vi "FT_Search All Select description.vi"(8 "error in (no error)":errorcluster, 11 "CTA Test#":string="CTA013A") -> (0 "error Out":errorcluster, 2 "All FT":T1(array[cluster]), 3 "Select Ft":T2)   [LabVIEW 2019]
uses:
  FT_Search all (state machine).ctl
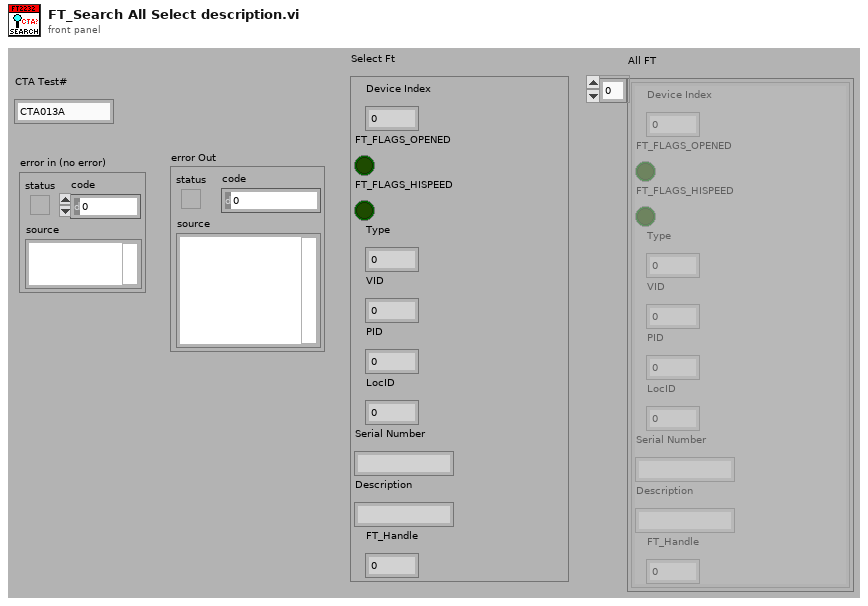
[diagram p1: front panel]
types:
  T1 = cluster{"Device Index":u32, "FT_FLAGS_OPENED":bool, "FT_FLAGS_HISPEED":bool, "Type":u32, "VID":u32, "PID":u32, "LocID":i32, "Serial Number":string, "Description":string, "FT_Handle":u32}[]
  T2 = cluster{"Device Index":u32, "FT_FLAGS_OPENED":bool, "FT_FLAGS_HISPEED":bool, "Type":u32, "VID":u32, "PID":u32, "LocID":i32, "Serial Number":string, "Description":string, "FT_Handle":u32}
  T3 = typedef "FT_Search all (state machine).ctl" = enum16{"Init", "Re_scan", "Close if Open", "Open FT", "Report FT", "Exit", "Error"}
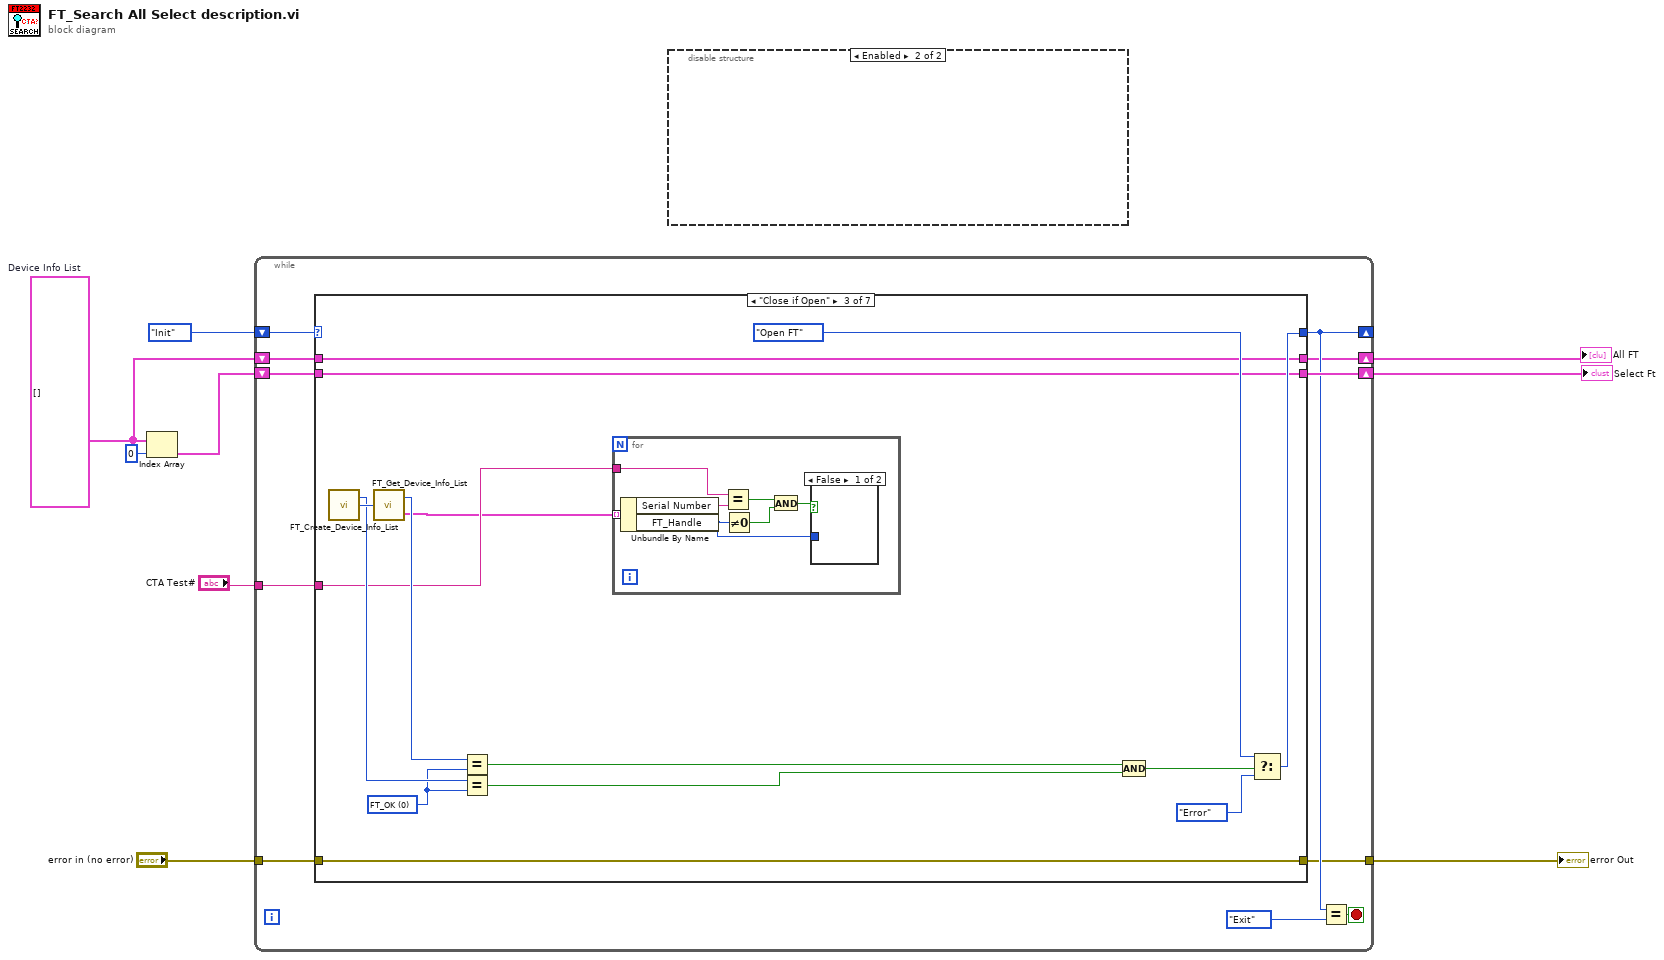
[diagram p0: block diagram]
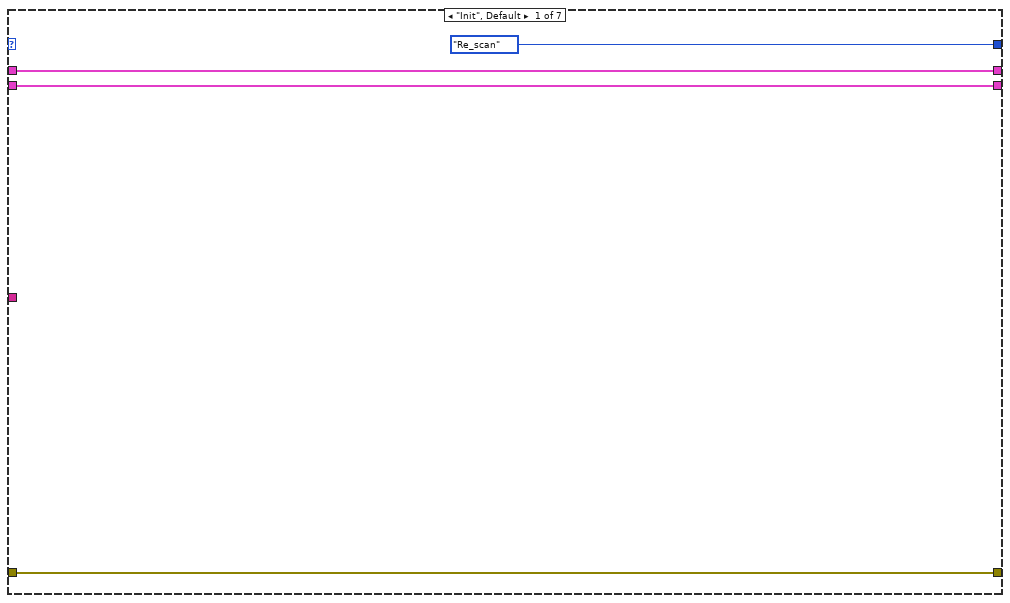
[diagram p3: hidden frame]
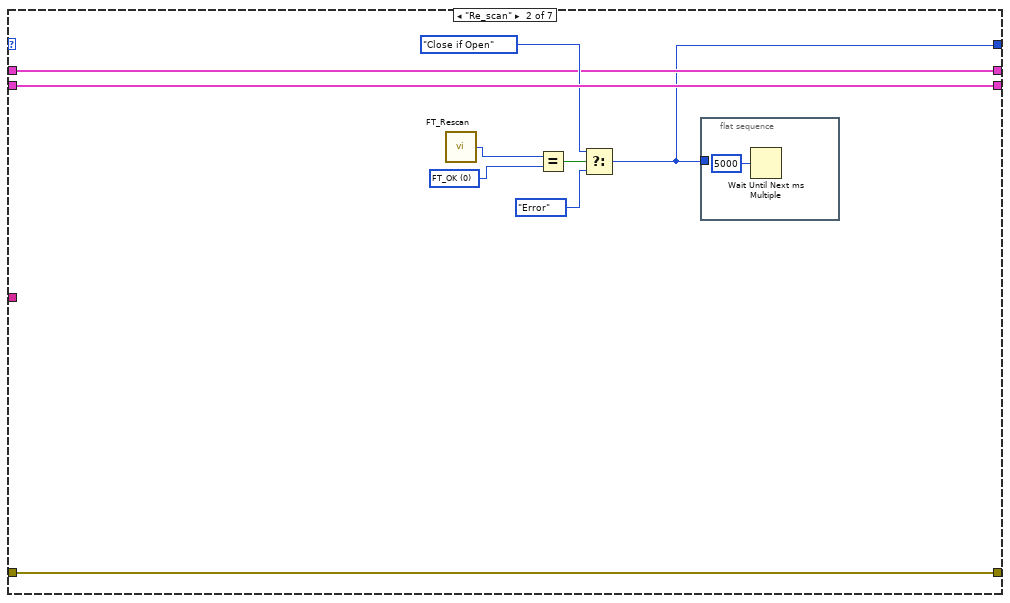
[diagram p4: hidden frame]
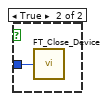
[diagram p5: hidden frame]
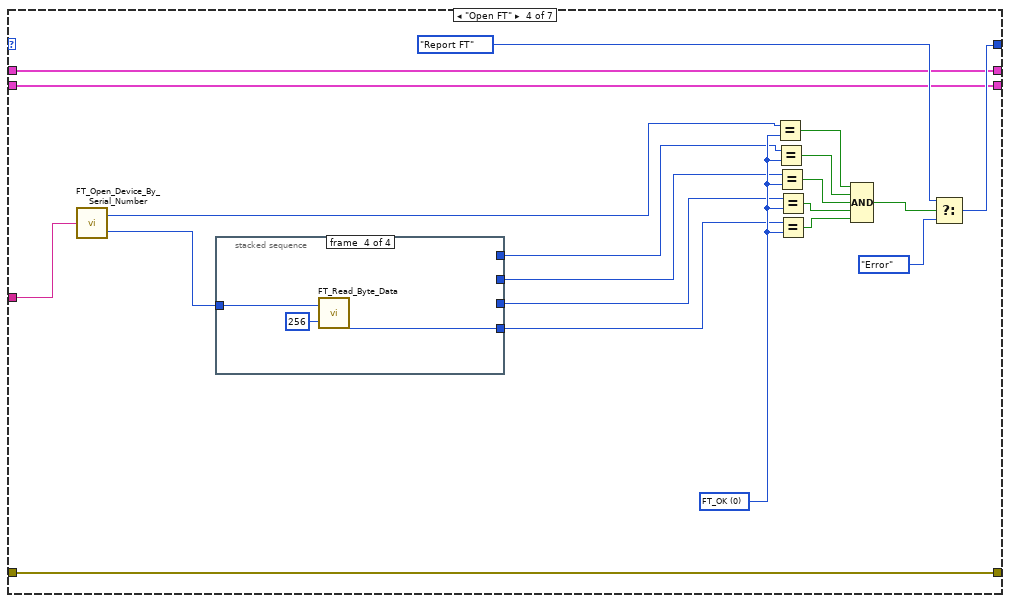
[diagram p6: hidden frame]
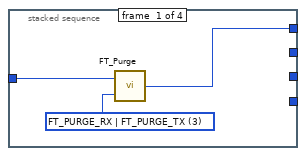
[diagram p7: hidden frame]
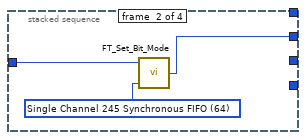
[diagram p8: hidden frame]
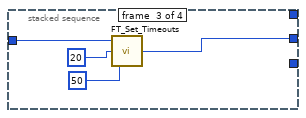
[diagram p9: hidden frame]
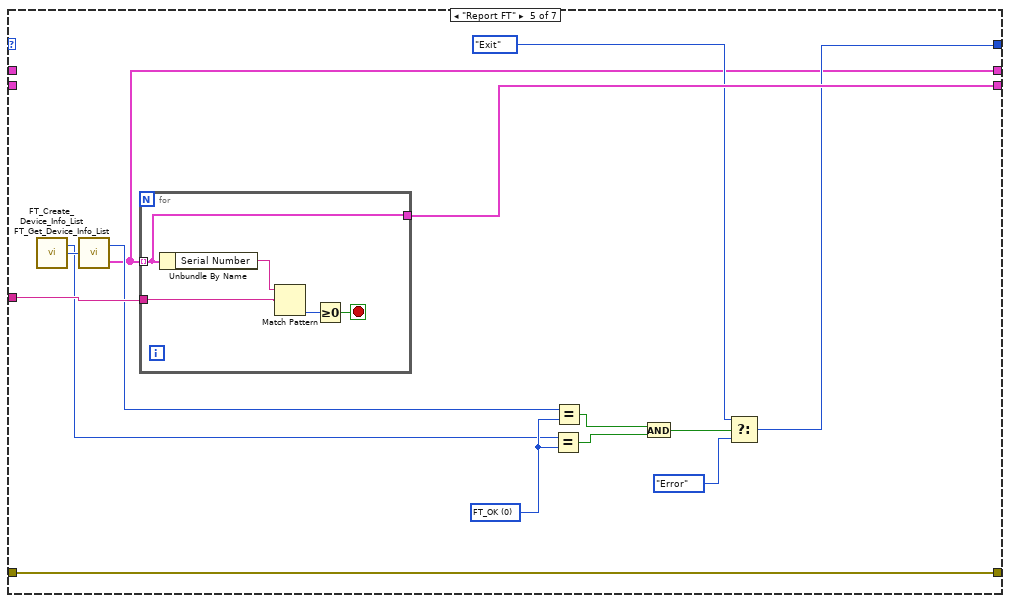
[diagram p10: hidden frame]
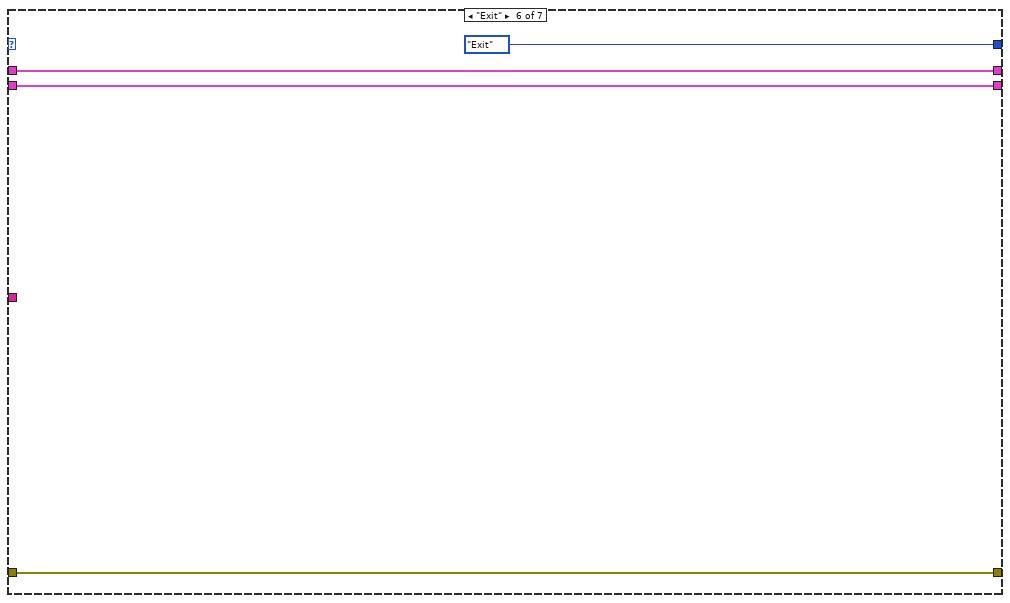
[diagram p11: hidden frame]
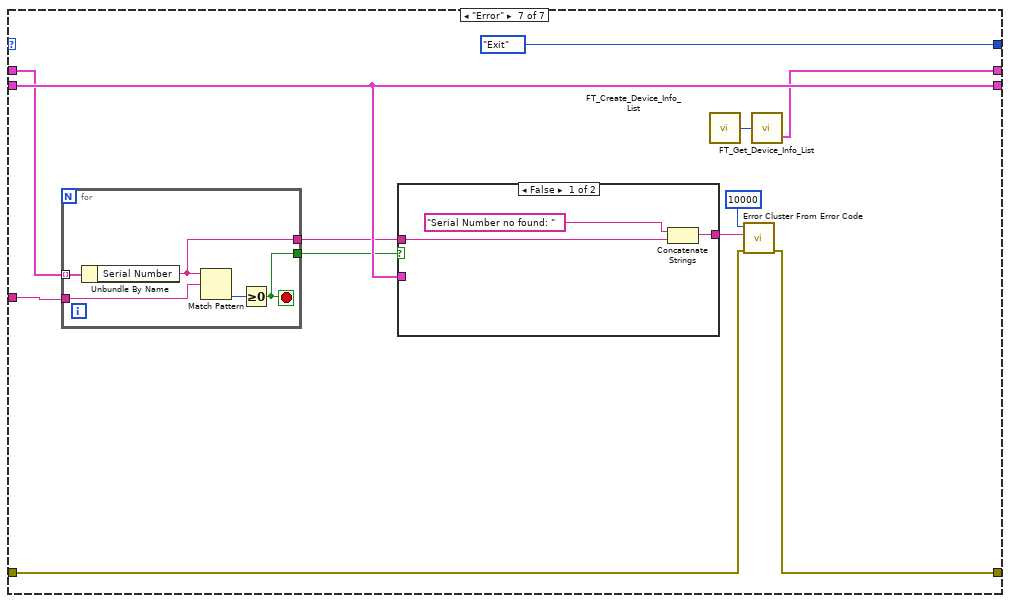
[diagram p12: hidden frame]
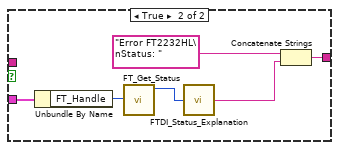
[diagram p13: hidden frame]
diagram:
  w3 = T1 []  # Device Info List
  n1 = Index Array(array=w3, index=0) -> (element=w6:T2)
  n2 = while {
    shift-right: [w15] -> _
    shift-left: FT_Search_all_(state_machine)."Init" ("State Search FT") -> [w20]
    tunnel: "CTA Test#" -> [w19]
    shift-right: [w16] -> w5
    shift-left: w6 -> [w18]
    tunnel: "error in (no error)" -> [w17]
    tunnel: [w12] -> w4
    shift-right: [w11] -> w2
    shift-left: w3 -> [w10]
    stop <- w13 stop-if-true
    n3 = case shown="\"Error\"" w20 {
      tunnel: w19 -> [_ _ w38 w65 w103 _ w118]
      tunnel: w18 -> [w24 w33 w35 w58 _ w113 w124]
      tunnel: w17 -> [w22 w32 w48 w77 w101 w111 w121]
      tunnel: [w24 w33 w35 w58 w102 w113 w124] -> w16
      tunnel: [FT_Search_all_(state_machine)."Re_scan" ("State Search FT") w25 w39 w67 w92 FT_Search_all_(state_machine)."Exit" ("State Search FT") FT_Search_all_(state_machine)."Exit" ("State Search FT")] -> w15
      tunnel: [w22 w32 w48 w77 w101 w111 w120] -> w12
      tunnel: [w21 w26 w37 w66 w91 w110 w114] -> w11
      tunnel: w10 -> [w21 w26 w37 w66 _ w110 w119]
      frame "Init", Default {
      }
      frame "Re_scan" {
        w31 = u32 0 items=["FT_OK", "FT_INVALID_HANDLE", "FT_DEVICE_NOT_FOUND", "FT_DEVICE_NOT_OPENED", "FT_IO_ERROR", "FT_INSUFFICIENT_RESOURCES", "FT_INVALID_PARAMETER", "FT_INVALID_BAUD_RATE", "FT_DEVICE_NOT_OPENED_FOR_ERASE", "FT_DEVICE_NOT_OPENED_FOR_WRITE", "FT_FAILED_TO_WRITE_DEVICE", "FT_EEPROM_READ_FAILED", "FT_EEPROM_WRITE_FAILED", "FT_EEPROM_ERASE_FAILED", "FT_EEPROM_NOT_PRESENT", "FT_EEPROM_NOT_PROGRAMMED", "FT_INVALID_ARGS", "FT_NOT_SUPPORTED", "FT_OTHER_ERROR"] ("FT_Status")
        n4 = call "FT_Rescan.vi"() -> ("FT_Status"=w30:u32)  [unwired: 1 in]
        n5 = Equal?(x=w30, y=w31) -> (x = y?=w29:bool)
        n6 = Select(t=FT_Search_all_(state_machine)."Close if Open" ("State Search FT"), s=w29, f=FT_Search_all_(state_machine)."Error") -> (s? t:f=w25:T3)
        n7 = flat-sequence {
          tunnel: w25 -> [_]
          frame #0 {
            n8 = Wait Until Next ms Multiple(millisecond multiple=u32 5000) -> ()  [unwired: 1 out]
          }
        }
      }
      frame "Close if Open" {
        w44 = u32 0 items=["FT_OK", "FT_INVALID_HANDLE", "FT_DEVICE_NOT_FOUND", "FT_DEVICE_NOT_OPENED", "FT_IO_ERROR", "FT_INSUFFICIENT_RESOURCES", "FT_INVALID_PARAMETER", "FT_INVALID_BAUD_RATE", "FT_DEVICE_NOT_OPENED_FOR_ERASE", "FT_DEVICE_NOT_OPENED_FOR_WRITE", "FT_FAILED_TO_WRITE_DEVICE", "FT_EEPROM_READ_FAILED", "FT_EEPROM_WRITE_FAILED", "FT_EEPROM_ERASE_FAILED", "FT_EEPROM_NOT_PRESENT", "FT_EEPROM_NOT_PROGRAMMED", "FT_INVALID_ARGS", "FT_NOT_SUPPORTED", "FT_OTHER_ERROR"] ("FT_Status")
        n9 = call "FT_Create_Device_Info_List.vi"() -> ("Number of Devices"=w49:u32, "FT_Status"=w46:u32)
        n10 = call "FT_Get_Device_Info_List.vi"("Number Of Devices"=w49) -> ("FT_Status"=w45:u32, "Device Info List"=w36:T1)
        n11 = Equal?(x=w45, y=w44) -> (x = y?=w43:bool)
        n12 = Equal?(x=w46, y=w44) -> (x = y?=w42:bool)
        n13 = for {
          tunnel: w36 -> [w56] mode=indexing
          tunnel: w38 -> [w55]
          n14 = Unbundle By Name(w56) -> ("Serial Number"=w50:string, "FT_Handle"=w51:u32)
          n15 = Equal?(x=w55, y=w50) -> (x = y?=w53:bool)
          n16 = Not Equal To 0?(x=w51) -> (x != 0?=w54:bool)
          n17 = And(x=w53, y=w54) -> (x .and. y?=w52:bool)
          n18 = case shown="False" w52 {
            tunnel: w51 -> [_ w57]
            frame False {
            }
            frame True {
              n19 = call "FT_Close_Device.vi"("Handle"=w57) -> ()  [unwired: 1 out]
            }
          }
        }
        n20 = Compound Arithmetic op=AND(w43, w42) -> (w41:bool)
        n21 = Select(t=FT_Search_all_(state_machine)."Open FT" ("State Search FT"), s=w41, f=FT_Search_all_(state_machine)."Error") -> (s? t:f=w39:T3)
      }
      frame "Open FT" {
        w76 = u32 0 items=["FT_OK", "FT_INVALID_HANDLE", "FT_DEVICE_NOT_FOUND", "FT_DEVICE_NOT_OPENED", "FT_IO_ERROR", "FT_INSUFFICIENT_RESOURCES", "FT_INVALID_PARAMETER", "FT_INVALID_BAUD_RATE", "FT_DEVICE_NOT_OPENED_FOR_ERASE", "FT_DEVICE_NOT_OPENED_FOR_WRITE", "FT_FAILED_TO_WRITE_DEVICE", "FT_EEPROM_READ_FAILED", "FT_EEPROM_WRITE_FAILED", "FT_EEPROM_ERASE_FAILED", "FT_EEPROM_NOT_PRESENT", "FT_EEPROM_NOT_PROGRAMMED", "FT_INVALID_ARGS", "FT_NOT_SUPPORTED", "FT_OTHER_ERROR"] ("FT_Status")
        n22 = call "FT_Open_Device_By_Serial_Number.vi"("Device Serial Number"=w65) -> ("FT_Status"=w63:u32, "Handle"=w64:u32)
        n23 = stacked-sequence {
          tunnel: w64 -> [w80 w82 w85 w90]
          tunnel: [w78 _ _ _] -> w62
          tunnel: [_ w81 _ _] -> w61
          tunnel: [_ _ w84 _] -> w60
          tunnel: [_ _ _ w88] -> w59
          frame #0 {
            w79 = u32 3 items=["FT_PURGE_RX"=1, "FT_PURGE_TX"=2, "FT_PURGE_RX | FT_PURGE_TX"=3] ("Purge Flags")
            n24 = call "FT_Purge.vi"("Purge Flags"=w79, "Handle"=w80) -> ("FT_Status"=w78:u32)
          }
          frame #1 {
            w83 = u8 64 items=["Reset Bit Mode"=0, "Asynchronous Bit Bang"=1, "MPSSE"=2, "Synchronous Bit Bang"=4, "MCU Host Bus Emulation"=8, "Fast Opto-Isolated Serial"=16, "CBUS Bit Bang"=32, "Single Channel 245 Synchronous FIFO"=64] ("Bit Mode")
            n25 = call "FT_Set_Bit_Mode.vi"("Bit Mode"=w83, "Handle"=w82) -> ("FT_Status"=w81:u32)  [unwired: 1 in]
          }
          frame #2 {
            n26 = call "FT_Set_Timeouts.vi"("Write Timeout"=u32 50, "Read Timeout"=u32 20, "Handle"=w85) -> ("FT_Status"=w84:u32)
          }
          frame #3 {
            n27 = call "FT_Read_Byte_Data.vi"("Handle"=w90, "Bytes To Read"=u32 256) -> ("FT_Status"=w88:u32)  [unwired: 2 out]
          }
        }
        n28 = Equal?(x=w63, y=w76) -> (x = y?=w75:bool)
        n29 = Equal?(x=w62, y=w76) -> (x = y?=w74:bool)
        n30 = Equal?(x=w61, y=w76) -> (x = y?=w73:bool)
        n31 = Equal?(x=w60, y=w76) -> (x = y?=w72:bool)
        n32 = Equal?(x=w59, y=w76) -> (x = y?=w71:bool)
        n33 = Compound Arithmetic op=AND(w75, w74, w73, w72, w71) -> (w69:bool)
        n34 = Select(t=FT_Search_all_(state_machine)."Report FT" ("State Search FT"), s=w69, f=FT_Search_all_(state_machine)."Error") -> (s? t:f=w67:T3)
      }
      frame "Report FT" {
        w100 = u32 0 items=["FT_OK", "FT_INVALID_HANDLE", "FT_DEVICE_NOT_FOUND", "FT_DEVICE_NOT_OPENED", "FT_IO_ERROR", "FT_INSUFFICIENT_RESOURCES", "FT_INVALID_PARAMETER", "FT_INVALID_BAUD_RATE", "FT_DEVICE_NOT_OPENED_FOR_ERASE", "FT_DEVICE_NOT_OPENED_FOR_WRITE", "FT_FAILED_TO_WRITE_DEVICE", "FT_EEPROM_READ_FAILED", "FT_EEPROM_WRITE_FAILED", "FT_EEPROM_ERASE_FAILED", "FT_EEPROM_NOT_PRESENT", "FT_EEPROM_NOT_PROGRAMMED", "FT_INVALID_ARGS", "FT_NOT_SUPPORTED", "FT_OTHER_ERROR"] ("FT_Status")
        n35 = call "FT_Create_Device_Info_List.vi"() -> ("Number of Devices"=w104:u32, "FT_Status"=w99:u32)
        n36 = call "FT_Get_Device_Info_List.vi"("Number Of Devices"=w104) -> ("FT_Status"=w98:u32, "Device Info List"=w91:T1)
        n37 = for {
          tunnel: w91 -> [w105] mode=indexing
          tunnel: w103 -> [w107]
          tunnel: [w105] -> w102
          stop <- w106 stop-if-true
          n38 = Unbundle By Name(w105) -> ("Serial Number"=w108:string)
          n39 = Match Pattern(string=w108, regular expression=w107) -> (offset past match=w109:i32)  [unwired: 4 out]
          n40 = Greater Or Equal To 0?(x=w109) -> (x >= 0?=w106:bool)
        }
        n41 = Equal?(x=w99, y=w100) -> (x = y?=w96:bool)
        n42 = Equal?(x=w98, y=w100) -> (x = y?=w97:bool)
        n43 = And(x=w97, y=w96) -> (x .and. y?=w94:bool)
        n44 = Select(t=FT_Search_all_(state_machine)."Exit" ("State Search FT"), s=w94, f=FT_Search_all_(state_machine)."Error") -> (s? t:f=w92:T3)
      }
      frame "Exit" {
      }
      frame "Error" {
        n45 = for {
          tunnel: w119 -> [w138] mode=indexing
          tunnel: w118 -> [w137]
          tunnel: [w136] -> w117
          tunnel: [w135] -> w116
          stop <- w136 stop-if-true
          n46 = Unbundle By Name(w138) -> ("Serial Number"=w135:string)
          n47 = Match Pattern(string=w135, regular expression=w137) -> (offset past match=w139:i32)  [unwired: 4 out]
          n48 = Greater Or Equal To 0?(x=w139) -> (x >= 0?=w136:bool)
        }
        n49 = case shown="False" w117 {
          tunnel: w124 -> [_ w134]
          tunnel: [w128 w130] -> w122
          tunnel: w116 -> [w126 _]
          frame False {
            n50 = Concatenate Strings("Serial Number no found: ", w126) -> (w128:string)
          }
          frame True {
            n51 = Unbundle By Name(w134) -> ("FT_Handle"=w133:u32)
            n52 = call "FT_Get_Status.vi"("Handle"=w133) -> ("FT_Status"=w131:u32)  [unwired: 3 out]
            n53 = call "FTDI_Status_Explanation.vi"("FT_Status"=w131) -> ("Status String"=w129:string)
            n54 = Concatenate Strings("Error FT2232HL\nStatus: ", w129) -> (w130:string)
          }
        }
        n55 = call "FT_Create_Device_Info_List.vi"() -> ("Number of Devices"=w115:u32)  [unwired: 1 out]
        n56 = call <vilib>:"Error Cluster From Error Code.vi"("error in (no error)"=w121, "error message (\"\")"=w122, "error code (0)"=10000 ("error code (no error:0)")) -> ("error out"=w120:errorcluster)  [unwired: 1 in, 5 out]
        n57 = call "FT_Get_Device_Info_List.vi"("Number Of Devices"=w115) -> ("Device Info List"=w114:T1)  [unwired: 1 out]
      }
    }
    n58 = Equal?(x=w15, y=FT_Search_all_(state_machine)."Exit" ("State Search FT")) -> (x = y?=w13:bool)
  }
  "Select Ft" <- w5
  "error Out" <- w4
  "All FT" <- w2
  n59 = disable-structure shown="Enabled" {
    frame Disabled {
    }
    frame Enabled {
    }
  }
